vi "Format Process Step Names.vi"(11 "Process Builder View in":refnum<class "Process Builder View.lvclass">) -> (3 "Process Builder View out":refnum<class "Process Builder View.lvclass">)   [LabVIEW 2019]
uses:
  <vilib>/gpm_packages/@cs/composed-car-wash/Source/Process Steps/Wait/Wait.lvclass
  <vilib>/gpm_packages/@cs/composed-car-wash/Source/Process Steps/Stop Under Body Wash/Stop Under Body Wash.lvclass
  <vilib>/gpm_packages/@cs/composed-car-wash/Source/Process Steps/Stop Tire Shine Foam/Stop Tire Shine Foam.lvclass
  <vilib>/gpm_packages/@cs/composed-car-wash/Source/Process Steps/Stop Spot Free Rinse/Stop Spot Free Rinse.lvclass
  <vilib>/gpm_packages/@cs/composed-car-wash/Source/Process Steps/Stop Pre-Soak/Stop Pre-Soak.lvclass
  <vilib>/gpm_packages/@cs/composed-car-wash/Source/Process Steps/Stop Low Pressure Wax/Stop Low Pressure Wax.lvclass
  <vilib>/gpm_packages/@cs/composed-car-wash/Source/Process Steps/Stop High Pressure Wash/Stop High Pressure Wash.lvclass
  <vilib>/gpm_packages/@cs/composed-car-wash/Source/Process Steps/Stop Bug Remover/Stop Bug Remover.lvclass
  <vilib>/gpm_packages/@cs/composed-car-wash/Source/Process Steps/Stop Air Dry/Stop Air Dry.lvclass
  <vilib>/gpm_packages/@cs/composed-car-wash/Source/Process Steps/Start Under Body Wash/Start Under Body Wash.lvclass
  <vilib>/gpm_packages/@cs/composed-car-wash/Source/Process Steps/Start Tire Shine Foam/Start Tire Shine Foam.lvclass
  <vilib>/gpm_packages/@cs/composed-car-wash/Source/Process Steps/Start Spot Free Rinse/Start Spot Free Rinse.lvclass
  <vilib>/gpm_packages/@cs/composed-car-wash/Source/Process Steps/Start Pre-Soak/Start Pre-Soak.lvclass
  <vilib>/gpm_packages/@cs/composed-car-wash/Source/Process Steps/Start Low Pressure Wax/Start Low Pressure Wax.lvclass
  <vilib>/gpm_packages/@cs/composed-car-wash/Source/Process Steps/Start High Pressure Wash/Start High Pressure Wash.lvclass
  <vilib>/gpm_packages/@cs/composed-car-wash/Source/Process Steps/Start Bug Remover/Start Bug Remover.lvclass
  <vilib>/gpm_packages/@cs/composed-car-wash/Source/Process Steps/Start Air Dry/Start Air Dry.lvclass
  <vilib>/gpm_packages/@cs/composed-car-wash/Source/Process Steps/Set Desired Station/Set Desired Station.lvclass
  <vilib>/gpm_packages/@cs/composed-car-wash/Source/Process Steps/Initialize HMI/Initialize HMI.lvclass
  <vilib>/gpm_packages/@cs/composed-car-wash/Source/iProcess Step Model/iProcess Step Model/iProcess Step Model.lvclass
  <vilib>/gpm_packages/@cs/composed-car-wash/Source/Process Steps/Exit/Exit.lvclass
  C:/Program Files/National Instruments/LabVIEW 2019/vi.lib/gpm_packages/@cs/composed-car-wash/Source/iProcess Step Model/iProcess Step Model/iProcess Step Model.lvclass
  C:/Program Files/National Instruments/LabVIEW 2019/vi.lib/gpm_packages/@cs/mva-core/Source/IModel/IModel/IModel.lvclass
  C:/Program Files/National Instruments/LabVIEW 2019/vi.lib/gpm_packages/@cs/mva-core/Source/IObserver/IObserver/IObserver.lvclass
  C:/Program Files/National Instruments/LabVIEW 2019/vi.lib/ActorFramework/Actor/Actor.lvclass
  <vilib>/gpm_packages/@cs/Test-executive-builder/Source/Test Executive Builder View/Test Executive Builder View/Test Executive Builder View.lvclass
  <vilib>/gpm_packages/@cs/composed-car-wash/Source/Process Builder View/Process Builder View.lvclass
  C:/Program Files/National Instruments/LabVIEW 2019/vi.lib/gpm_packages/@cs/Test-executive-builder/Source/Test Executive Builder View/Test Executive Builder View/Test Executive Builder View.lvclass
  C:/Program Files/National Instruments/LabVIEW 2019/vi.lib/gpm_packages/@cs/mva-viewable/Source/IViewable/IViewable/IViewable.lvclass
  C:/Program Files/National Instruments/LabVIEW 2019/vi.lib/gpm_packages/@cs/mva-viewable/Source/ActorEvents/IEventAggregator/IEventAggregator.lvclass
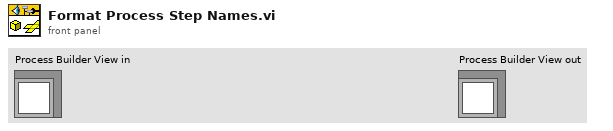
[diagram p1: front panel]
types:
  T1 = cluster{refnum<class "iProcess Step Model.lvclass">[]}
  T2 = cluster{refnum<class "iProcess Step Model.lvclass">[]}[]
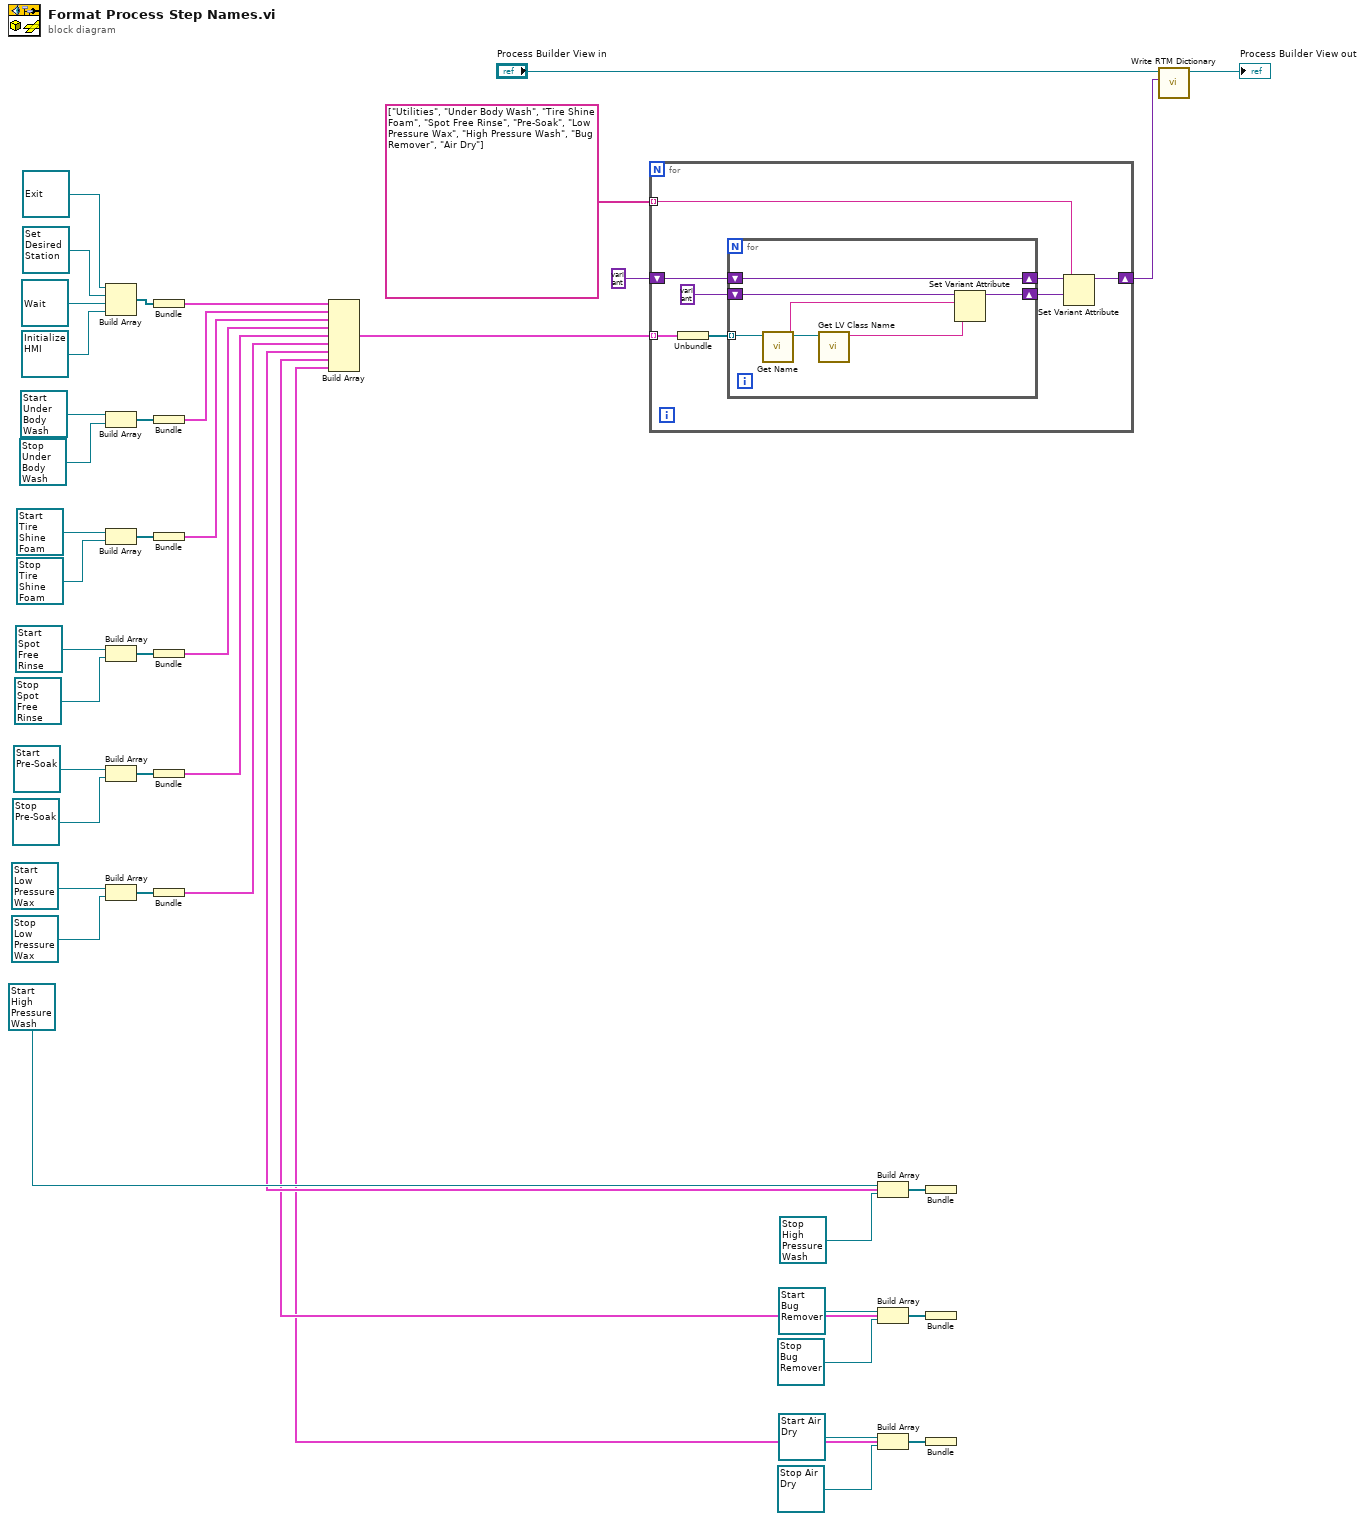
[diagram p0: block diagram]
diagram:
  n1 = Build Array(refnum<class "Exit.lvclass"> refnum ("Exit.lvclass"), refnum<class "Set Desired Station.lvclass"> refnum ("Set Desired Station.lvclass"), refnum<class "Wait.lvclass"> refnum ("Wait.lvclass"), refnum<class "Initialize HMI.lvclass"> refnum ("Initialize HMI.lvclass")) -> (w40:refnum<class "iProcess Step Model.lvclass">[])
  n2 = Build Array(refnum<class "Start Under Body Wash.lvclass"> refnum ("Start Under Body Wash.lvclass"), refnum<class "Stop Under Body Wash.lvclass"> refnum ("Stop Under Body Wash.lvclass")) -> (w39:refnum<class "iProcess Step Model.lvclass">[])
  n3 = Build Array(refnum<class "Start Tire Shine Foam.lvclass"> refnum ("Start Tire Shine Foam.lvclass"), refnum<class "Stop Tire Shine Foam.lvclass"> refnum ("Stop Tire Shine Foam.lvclass")) -> (w36:refnum<class "iProcess Step Model.lvclass">[])
  n4 = Build Array(refnum<class "Start Spot Free Rinse.lvclass"> refnum ("Start Spot Free Rinse.lvclass"), refnum<class "Stop Spot Free Rinse.lvclass"> refnum ("Stop Spot Free Rinse.lvclass")) -> (w33:refnum<class "iProcess Step Model.lvclass">[])
  n5 = Build Array(refnum<class "Start Pre-Soak.lvclass"> refnum ("Start Pre-Soak.lvclass"), refnum<class "Stop Pre-Soak.lvclass"> refnum ("Stop Pre-Soak.lvclass")) -> (w30:refnum<class "iProcess Step Model.lvclass">[])
  n6 = Build Array(refnum<class "Start Low Pressure Wax.lvclass"> refnum ("Start Low Pressure Wax.lvclass"), refnum<class "Stop Low Pressure Wax.lvclass"> refnum ("Stop Low Pressure Wax.lvclass")) -> (w26:refnum<class "iProcess Step Model.lvclass">[])
  n7 = Bundle(w40) -> (w14:T1)  [unwired: 1 in]
  n8 = Bundle(w39) -> (w13:T1)  [unwired: 1 in]
  n9 = Bundle(w36) -> (w12:T1)  [unwired: 1 in]
  n10 = Bundle(w33) -> (w11:T1)  [unwired: 1 in]
  n11 = Bundle(w30) -> (w10:T1)  [unwired: 1 in]
  n12 = Bundle(w26) -> (w9:T1)  [unwired: 1 in]
  n13 = Build Array(refnum<class "Start High Pressure Wash.lvclass"> refnum ("Start High Pressure Wash.lvclass"), refnum<class "Stop High Pressure Wash.lvclass"> refnum ("Stop High Pressure Wash.lvclass")) -> (w23:refnum<class "iProcess Step Model.lvclass">[])
  n14 = Build Array(refnum<class "Start Bug Remover.lvclass"> refnum ("Start Bug Remover.lvclass"), refnum<class "Stop Bug Remover.lvclass"> refnum ("Stop Bug Remover.lvclass")) -> (w20:refnum<class "iProcess Step Model.lvclass">[])
  n15 = Build Array(refnum<class "Start Air Dry.lvclass"> refnum ("Start Air Dry.lvclass"), refnum<class "Stop Air Dry.lvclass"> refnum ("Stop Air Dry.lvclass")) -> (w17:refnum<class "iProcess Step Model.lvclass">[])
  n16 = Bundle(w23) -> (w8:T1)  [unwired: 1 in]
  n17 = Bundle(w20) -> (w7:T1)  [unwired: 1 in]
  n18 = Bundle(w17) -> (w6:T1)  [unwired: 1 in]
  n19 = Build Array(w14, w13, w12, w11, w10, w9, w8, w7, w6) -> (w3:T2)
  n20 = for {
    tunnel: string[] ["Utilities", "Under Body Wash", "Tire Shine Foam", "Spot Free Rinse", "Pre-Soak", "Low Pressure Wax", "High Pressure Wash", "Bug Remover", "Air Dry"] -> [w49] mode=indexing
    shift-right: [w50] -> w2
    shift-left: variant -> [w52]
    tunnel: w3 -> [w46] mode=indexing
    n21 = Unbundle(w46) -> (w45:refnum<class "iProcess Step Model.lvclass">[])
    n22 = for {
      shift-right: [w57] -> w51
      shift-left: w52 -> [w57]
      shift-right: [w58] -> w47
      shift-left: variant -> [w59]
      tunnel: w45 -> [w55] mode=indexing
      n23 = call <vilib>:"Get Name.vi"("iProcess Step Model in"=w55) -> ("Name"=w53:string, "iProcess Step Model out"=w54:refnum<class "iProcess Step Model.lvclass">)  [unwired: 9 in]
      n24 = call <vilib>:"Get LV Class Name.vi"("object"=w54) -> ("class name"=w56:string)  [unwired: 9 in, 1 out]
      n25 = Set Variant Attribute(Variant=w59, name=w53, value=w56) -> (Variant out=w58:variant)  [unwired: 1 in, 2 out]
    }
    n26 = Set Variant Attribute(Variant=w51, name=w49, value=w47) -> (Variant out=w50:variant)  [unwired: 1 in, 2 out]
  }
  n27 = call <vilib>:"Write RTM Dictionary.vi"("RTM Dictionary"=w2, "Test Executive Builder View in"="Process Builder View in") -> ("Test Executive Builder View out"=→"Process Builder View out":refnum<class "Process Builder View.lvclass">)  [unwired: 9 in]
